vi "Save Recall Setup.vi"(8 "error in (no error)":errorcluster, 10 "Action Type (0: Save Present Setup)":i32(ring) items=["Save Present Setup", "Recall Saved Setup"], 11 "VISA resource name":refnum<visa-resource-name>) -> (0 "error out":errorcluster, 3 "VISA resource name out":refnum<visa-resource-name>)   [LabVIEW 2011, in "Keithley 2182.lvlib"]
doc: "Saves instrument's present setup or Recalls saved setup."
uses:
  Keithley 2182.lvlib
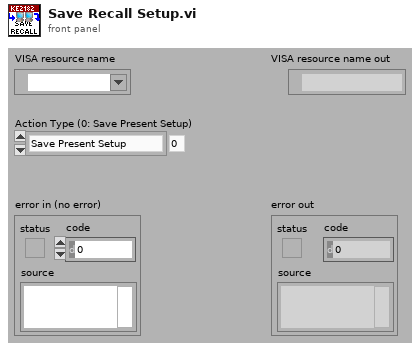
[diagram p1: front panel]
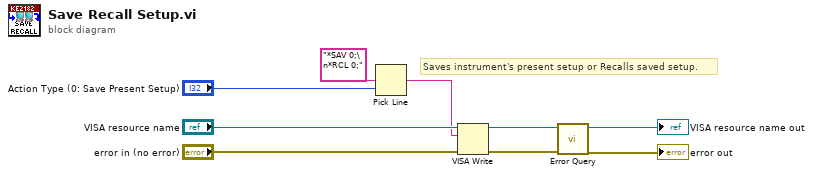
[diagram p0: block diagram]
diagram:
  # "Saves instrument's present setup or Recalls saved setup."
  n1 = Pick Line(multi-line string="*SAV 0;\n*RCL 0;", line index="Action Type (0: Save Present Setup)") -> (output string=w3:string)  [unwired: 1 in]
  n2 = VISA Write(VISA resource name="VISA resource name", write buffer=w3, error in (no error)="error in (no error)") -> (VISA resource name out=w7:refnum<visa-resource-name>, error out=w6:errorcluster)  [unwired: 1 out]
  n3 = call "Error Query.vi"("error in (no error)"=w6, "VISA resource name"=w7) -> ("error out"=→"error out":errorcluster, "VISA resource name out"=→"VISA resource name out":refnum<visa-resource-name>)  [unwired: 6 in, 2 out]
